vi "set time.vi"(8 "error in":errorcluster, 9 "New DateTime":timestamp, 11 "Path":path) -> (0 "error out":errorcluster)   [LabVIEW 2023, in "EXIF Modifier.lvlib"]
uses:
  EXIF Modifier.lvlib
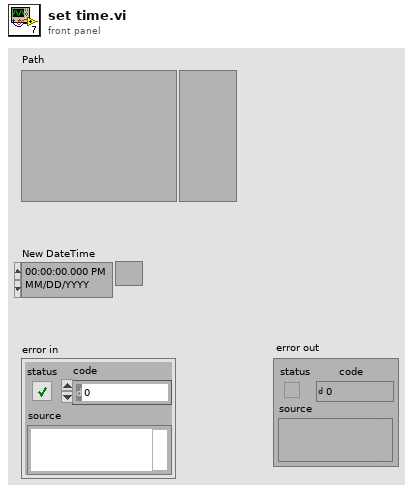
[diagram p1: front panel]
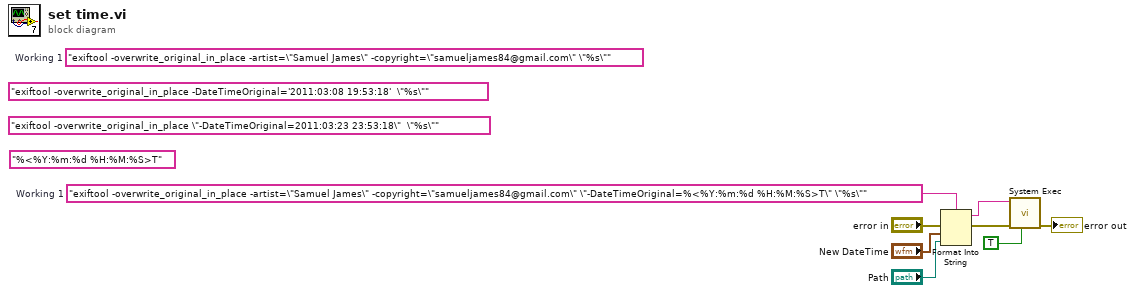
[diagram p0: block diagram]
diagram:
  (unwired) "%<%Y:%m:%d %H:%M:%S>T" ("format string")
  (unwired) "exiftool -overwrite_original_in_place -artist=\"Samuel James\" -copyright=\"samueljames84@gmail.com\" \"%s\""  # Working 1
  w6 = "exiftool -overwrite_original_in_place -artist=\"Samuel James\" -copyright=\"samueljames84@gmail.com\" \"-DateTimeOriginal=%<%Y:%m:%d %H:%M:%S>T\" \"%s\""  # Working 1
  (unwired) "exiftool -overwrite_original_in_place -DateTimeOriginal='2011:03:08 19:53:18'  \"%s\"" ("command line")
  (unwired) "exiftool -overwrite_original_in_place \"-DateTimeOriginal=2011:03:23 23:53:18\"  \"%s\"" ("command line")
  n1 = Format Into String(format string=w6, error in="error in", "New DateTime", "Path") -> (resulting string=w7:string, error out=w3:errorcluster)  [unwired: 1 in]
  n2 = call <vilib>:"System Exec.vi"("run minimized? (F)"=TRUE, "error in (no error)"=w3, "command line"=w7) -> ("error out"=→"error out":errorcluster)  [unwired: 5 in, 3 out]
